vi "close_connection.vi"(0 "reference":i32, 11 "error in (no error)":errorcluster) -> (15 "error out":errorcluster)   [LabVIEW 2012]
doc: "Closes the reference to the specified device.\n\nImplementss the USB Communication API function \"fnPerformaxComClose()'.\n\nProduced By:\n\nChristopher Lemieux\nKod Integrations, LLC\n4835 Marianne Drive\nMount Airy, MD 21771\nhttp://www.kodintegrations.com\nemail: clemieux@kodintegrations.com\nphone: (240) 687-1288"
uses:
  support/controls/errors_actions.ctl
  PerformaxCom.dll
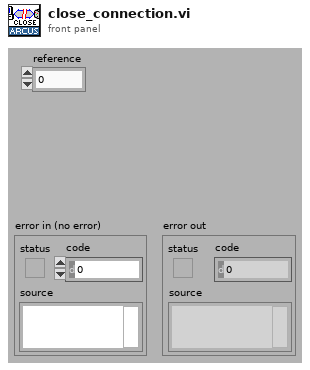
[diagram p1: front panel]
types:
  T1 = typedef "errors_actions.ctl" = enum16{"clearBuff", "closeRef", "noDeviceInfo", "noDevices", "openRef", "sendReceive", "setTimeouts", "unknown"}
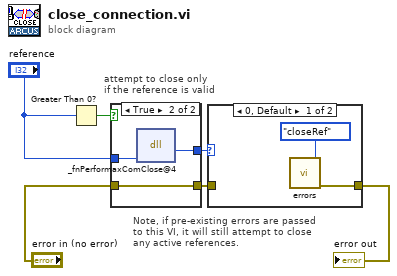
[diagram p0: block diagram]
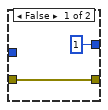
[diagram p2: hidden frame]
diagram:
  # "Note, if pre-existing errors are passed\nto this VI, it will still attempt to close\nany active references."
  # "attempt to close only\nif the reference is valid"
  n1 = Greater Than 0?(x="reference") -> (x > 0?=w2:bool)
  n2 = case shown="True" w2 {
    tunnel: [1 w11] -> w4
    tunnel: [w7 w10] -> w3
    tunnel: "error in (no error)" -> [w7 w10]
    tunnel: "reference" -> [_ w9]
    frame False {
    }
    frame True {
      n3 = dll-call lib="PerformaxCom.dll" fn="_fnPerformaxComClose@4"("reference"=w9) -> (w11:i32)  [unwired: 4 in, 2 out]
    }
  }
  n4 = case shown="0, Default" w4 {
    tunnel: [w12 w14] -> w5
    tunnel: w3 -> [_ w14]
    frame 0, Default {
      n5 = call "errors.vi"("errors"=errors_actions."closeRef") -> ("error out"=w12:errorcluster)  [unwired: 14 in]
    }
    frame 1 {
    }
  }
  "error out" <- w5
